vi "Selecao.View.vi"() -> ()   [LabVIEW 2019]
uses:
  Telas.ctl
  <vilib>/Utility/miscctls.llb/LVPositionTypeDef.ctl
  <vilib>/Utility/miscctls.llb/LVPointTypeDef.ctl
panel:
  out "ProximaTela":T1
  in  "Tab":enum32{"Page 1", "Page 2"}(tab)
  in  "ParametrosMedicao":bool
  in  "Medicao":bool
  in  "Config":bool
  in  "Parar":bool
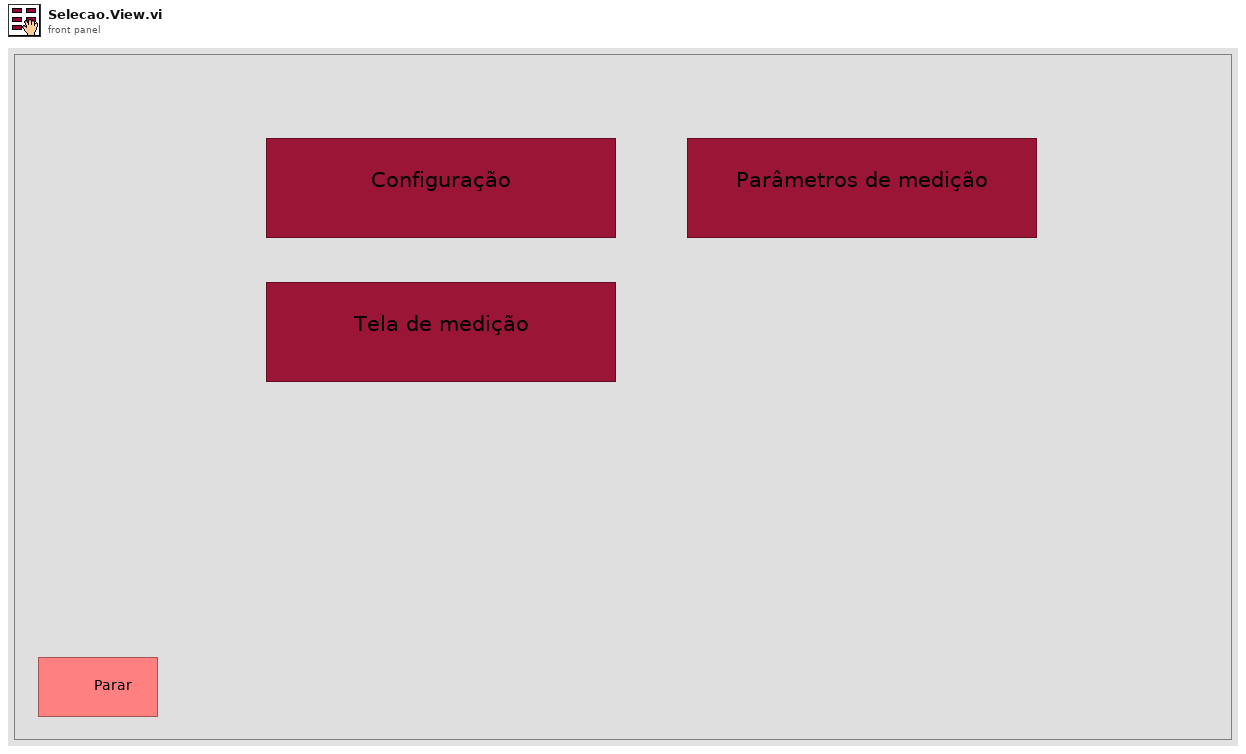
[diagram p1: front panel]
types:
  T1 = typedef "Telas.ctl" = enum16{"Selecao", "Config", "Medicao"}
  T2 = typedef "LVPositionTypeDef.ctl" = cluster{"Left":i32, "Top":i32}
  T3 = typedef "LVPointTypeDef.ctl" = cluster{"Horizontal":i16, "Vertical":i16}
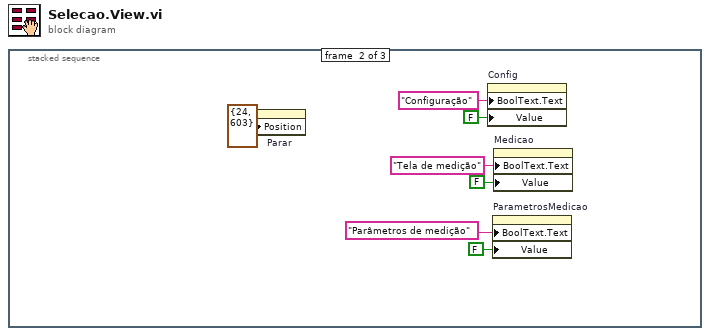
[diagram p0: block diagram]
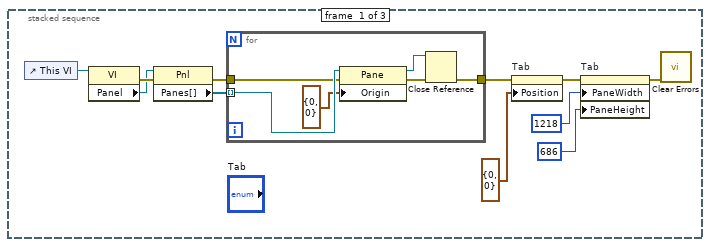
[diagram p2: hidden frame]
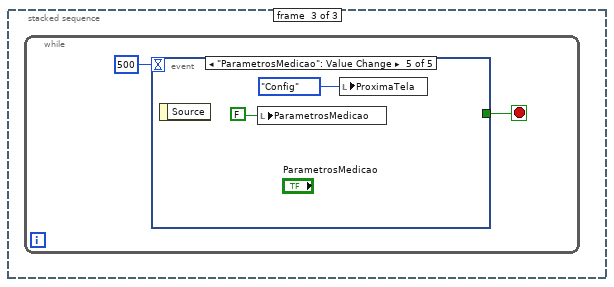
[diagram p3: hidden frame]
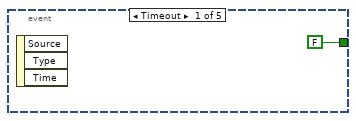
[diagram p4: hidden frame]
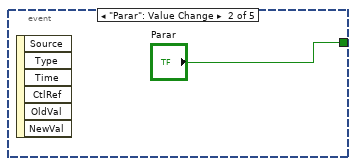
[diagram p5: hidden frame]
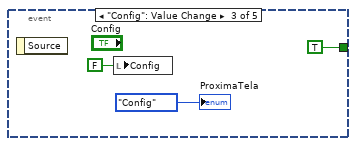
[diagram p6: hidden frame]
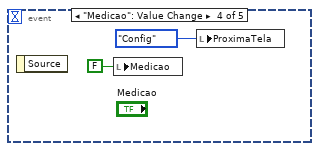
[diagram p7: hidden frame]
diagram:
  n1 = stacked-sequence {
    frame #0 {
      n2 = control-ref of="This VI"() -> (w8:refnum<vi>)
      n3 = property class="VI"(reference=w8) -> (error out=w11:errorcluster, "Panel"=w10:refnum<vi>)  [unwired: 1 in, 1 out]
      n4 = property class="Pnl"(reference=w10, error in=w11) -> (error out=w7:errorcluster, "Panes[]"=w9:refnum<vi>[])  [unwired: 1 out]
      n5 = for {
        tunnel: w9 -> [w17] mode=indexing
        tunnel: w7 -> [w13]
        tunnel: [w12] -> w6
        n6 = property class="Pane"(reference=w17, error in=w13, "Origin"=T3 {"Horizontal"=0, "Vertical"=0}) -> (reference out=w14:refnum<vi>, error out=w15:errorcluster)
        n7 = Close Reference(reference=w14, error in (no error)=w15) -> (error out=w12:errorcluster)
      }
      n8 = property on="Tab" class="TabCtl (strict)"(error in=w6, "Position"=T2 {"Left"=0, "Top"=0}) -> (error out=w2:errorcluster)  [unwired: 1 in, 1 out]
      n9 = property on="Tab" class="TabCtl (strict)"(error in=w2, "PaneWidth"=u32 1218 ("Tab Control Pane Dimension:Width"), "PaneHeight"=u32 686 ("Tab Control Pane Dimension:Height")) -> (error out=w1:errorcluster)  [unwired: 1 in, 1 out]
      n10 = call <vilib>:"Clear Errors.vi"("error in (no error)"=w1) -> ()  [unwired: 5 in, 2 out]
    }
    frame #1 {
      n11 = property on="Parar" class="Bool"("Position"=T2 {"Left"=24, "Top"=603}) -> ()  [unwired: 2 in, 2 out]
      n12 = property on="Config" class="Bool (strict)"("BoolText.Text"="Configuração" ("Boolean Text.Text"), "Value"=FALSE ("Config")) -> ()  [unwired: 2 in, 2 out]
      n13 = property on="ParametrosMedicao" class="Bool (strict)"("BoolText.Text"="Parâmetros de medição" ("Boolean Text.Text"), "Value"=FALSE ("ParametrosMedicao")) -> ()  [unwired: 2 in, 2 out]
      n14 = property on="Medicao" class="Bool (strict)"("BoolText.Text"="Tela de medição" ("Boolean Text.Text"), "Value"=FALSE ("Medicao")) -> ()  [unwired: 2 in, 2 out]
    }
    frame #2 {
      n15 = while {
        stop <- w25 stop-if-true
        n16 = event shown="[4] \"ParametrosMedicao\": Value Change" {
          selector: _ -> [_ _ _ _ _]
          dyn-events: _ -> [_ _ _ _ _]
          timeout: 500 -> [_ _ _ _ _]
          tunnel: [FALSE "Parar" TRUE ("stop") _ _] -> w25
          event Timeout {
            n17 = event-data() -> ()  [unwired: 1 in, 3 out]
          }
          event "Parar": Value Change {
            n18 = event-data() -> ()  [unwired: 1 in, 6 out]
          }
          event "Config": Value Change {
            n19 = event-data() -> ()  [unwired: 1 in, 1 out]
            n20 = local write "Config"(FALSE ("Config")) -> ()
            "ProximaTela" <- Telas."Config" ("NextScreen")
          }
          event "Medicao": Value Change {
            n21 = event-data() -> ()  [unwired: 1 in, 1 out]
            n22 = local write "Medicao"(FALSE ("Medicao")) -> ()
            n23 = local write "ProximaTela"(Telas."Config" ("NextScreen")) -> ()
          }
          event "ParametrosMedicao": Value Change {
            n24 = event-data() -> ()  [unwired: 1 in, 1 out]
            n25 = local write "ParametrosMedicao"(FALSE ("Medicao")) -> ()
            n26 = local write "ProximaTela"(Telas."Config" ("NextScreen")) -> ()
          }
        }
      }
    }
  }
